vi "写入SN.vi"(8 "error in":errorcluster, 9 "流水号":string, 10 "产品料号":string, 11 "产品名":string) -> (0 "error out":errorcluster, 2 "return":i32)   [LabVIEW 2016]
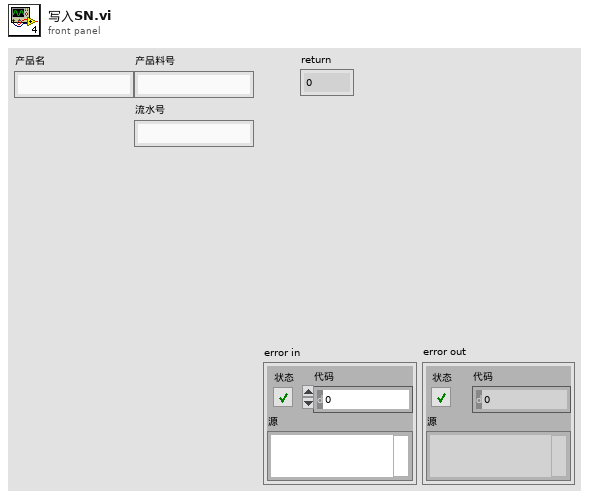
[diagram p1: front panel]
types:
  T1 = cluster{"byCmdType":u8, "bySubCmd":u8, "byPara":u8, "byAddr_h":u8, "byAddr_l":u8, "byAddr_ll":u8, "byLen_h":u8, "byLen_l":u8}
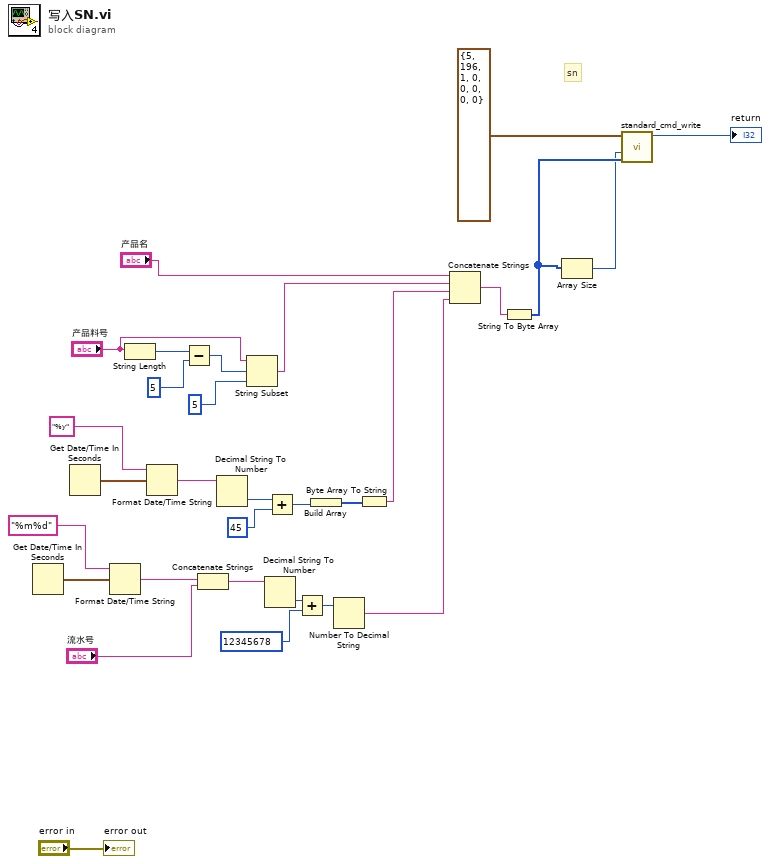
[diagram p0: block diagram]
diagram:
  # "sn"
  n1 = Get Date/Time In Seconds() -> (seconds since 1Jan1904=w26:timestamp)
  n2 = Get Date/Time In Seconds() -> (seconds since 1Jan1904=w29:timestamp)
  n3 = Format Date/Time String(time format string (%c)="%m%d", seconds (now)=w26) -> (date/time string=w3:string)  [unwired: 1 in]
  n4 = String Length(string="产品料号") -> (length=w12:i32)
  n5 = Format Date/Time String(time format string (%c)="%y", seconds (now)=w29) -> (date/time string=w25:string)  [unwired: 1 in]
  n6 = Subtract(x=w12, y=5 ("length (rest)")) -> (x-y=w10:i32)
  n7 = Concatenate Strings(w3, "流水号") -> (w7:string)
  n8 = Decimal String To Number(string=w25) -> (number=w24:i32)  [unwired: 2 in, 1 out]
  n9 = String Subset(string="产品料号", offset (0)=w10, length (rest)=5 ("length (rest)")) -> (substring=w8:string)
  n10 = Decimal String To Number(string=w7) -> (number=w6:i32)  [unwired: 2 in, 1 out]
  n11 = Add(x=w24, y=45) -> (x+y=w22:i32)
  n12 = Add(x=w6, y=12345678) -> (x+y=w4:i32)
  n13 = Build Array(w22) -> (w21:i32[])
  n14 = Number To Decimal String(number=w4) -> (decimal integer string=w1:string)  [unwired: 1 in]
  n15 = Byte Array To String(unsigned byte array=w21) -> (string=w19:string)
  n16 = Concatenate Strings("产品名", w8, w19, w1) -> (w18:string)
  n17 = String To Byte Array(string=w18) -> (unsigned byte array=w17:u8[])
  n18 = Array Size(array=w17) -> (size(s)=w16:i32)
  n19 = call "standard_cmd_write.vi"("data"=w17, "dwLen"=w16, "cmd_std_header_t"=T1 {"byCmdType"=5, "bySubCmd"=196, "byPara"=1, "byAddr_h"=0, "byAddr_l"=0, "byAddr_ll"=0, "byLen_h"=0, "byLen_l"=0}) -> ("return"=→"return":i32)  [unwired: 7 in, 1 out]
  "error out" <- "error in"
